vi "ShowOtherMsg.vi"(0 "影像处理无异常":bool, 1 "显示消息":string, 2 "引用句柄输入":T1) -> ()   [LabVIEW 2014]
uses:
  <vilib>/vision/Image Controls.llb/IMAQ Image.ctl
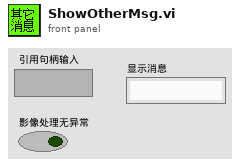
[diagram p1: front panel]
types:
  T1 = typedef "IMAQ Image.ctl" = refnum<image>
  T2 = cluster{"Desired Font (Application)":enum16{"User-specified Font", "Application Font", "System Font", "Dialog Font"}, "[User-specified Font]":cluster{"Font Name":string, "Size":i16, "Strikeout?":bool, "Italic?":bool, "Underline?":bool, "Outline?":bool, "Shadow?":bool, "Bold?":bool, "Rotation Angle":dbl}, "Horizontal Alignment":i16, "Vertical Alignment":i16}
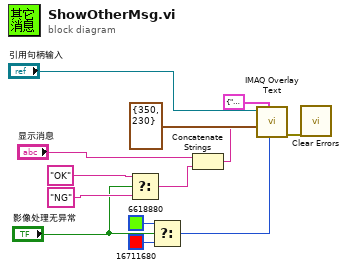
[diagram p0: block diagram]
diagram:
  n1 = Select(t="OK", s="影像处理无异常", f="NG") -> (s? t:f=w5:string)
  n2 = Select(t=u32 6618880 ("Text Color (black)"), s="影像处理无异常", f=u32 16711680 ("Text Color (black)")) -> (s? t:f=w1:u32)
  n3 = Concatenate Strings("显示消息", w5) -> (w6:string)
  n4 = call "IMAQ Overlay Text"("Text Color (black)"=w1, "Font, Size & Style"=T2 {"Desired Font (Application)"=enum."User-specified Font", "[User-specified Font]"={"Font Name"="", "Size"=150, "Strikeout?"=FALSE, "Italic?"=FALSE, "Underline?"=FALSE, "Outline?"=FALSE, "Shadow?"=FALSE, "Bold?"=TRUE, "Rotation Angle"=0.0}, "Horizontal Alignment"=0, "Vertical Alignment"=0}, "String"=w6, "Origin"=cluster{"X":i32, "Y":i32} {"X"=350, "Y"=230}, "Image"="引用句柄输入") -> ("error out"=w12:errorcluster)  [unwired: 5 in, 1 out]
  n5 = call <vilib>:"Clear Errors.vi"("error in (no error)"=w12) -> ()  [unwired: 5 in, 2 out]
